vi "toml_string_join.vi"(7 "separator (,)":string=",", 11 "strings":string[](array[string])) -> (3 "string":string)   [LabVIEW 2017]
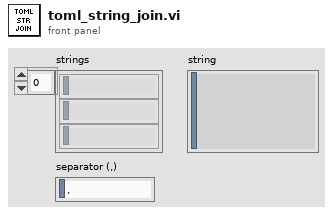
[diagram p1: front panel]
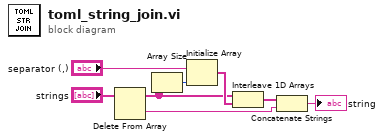
[diagram p0: block diagram]
diagram:
  n1 = Delete From Array(array="strings") -> (deleted portion=w2:string, array with subset deleted=w4:string[])  [unwired: 2 in]
  n2 = Array Size(array=w4) -> (size(s)=w7:i32)
  n3 = Initialize Array("separator (,)", w7) -> (w5:string[])
  n4 = Interleave 1D Arrays(w4, w5) -> (w3:string[])
  n5 = Concatenate Strings(w3, w2) -> (→"string":string)
